vi "readIUPfromTP.vi"(0 "HEX String to Decode":string) -> (1 "Numeric":dbl, 2 "Numeric 2":dbl, 3 "Numeric 3":dbl)   [LabVIEW 2015]
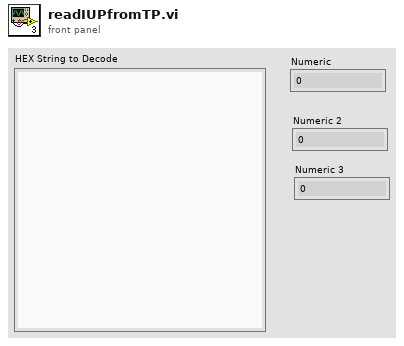
[diagram p1: front panel]
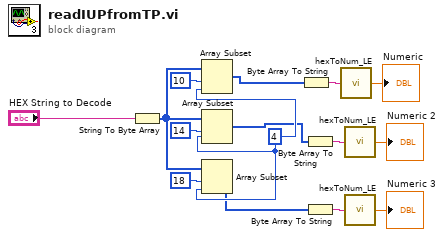
[diagram p0: block diagram]
diagram:
  w7 = 4 ("length")
  n1 = String To Byte Array(string="HEX String to Decode") -> (unsigned byte array=w10:u8[])
  n2 = Array Subset(array=w10, index=10, length=w7) -> (w13:u8[])
  n3 = Array Subset(array=w10, index=14, length=w7) -> (w4:u8[])
  n4 = Array Subset(array=w10, index=18, length=w7) -> (w2:u8[])
  n5 = Byte Array To String(unsigned byte array=w13) -> (string=w12:string)
  n6 = Byte Array To String(unsigned byte array=w4) -> (string=w3:string)
  n7 = Byte Array To String(unsigned byte array=w2) -> (string=w1:string)
  n8 = call "hexToNum_LE.vi"("String"=w12) -> ("Numeric"=→"Numeric":dbl)
  n9 = call "hexToNum_LE.vi"("String"=w3) -> ("Numeric"=→"Numeric 2":dbl)
  n10 = call "hexToNum_LE.vi"("String"=w1) -> ("Numeric"=→"Numeric 3":dbl)
